vi "Get MeasLink API Path.vi"(11 "error in (no error)":errorcluster) -> (6 "MeasLink API Paths":path[](array[path]), 15 "error out":errorcluster)   [LabVIEW 2021, in "Path Functions.lvlib"]
uses:
  Path Functions.lvlib
  Converter Reusables/Converter Reusables.lvlib
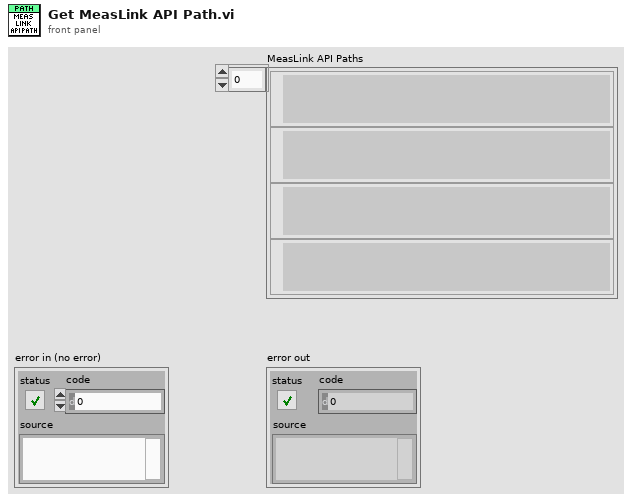
[diagram p1: front panel]
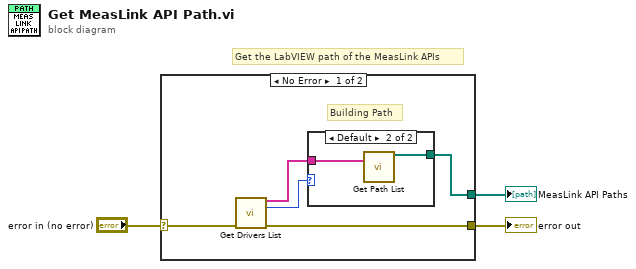
[diagram p0: block diagram]
diagram:
  # "Get the LabVIEW path of the MeasLink APIs"
  n1 = case shown="No Error" "error in (no error)" {
    selector: "error in (no error)" -> [w4 w11]
    tunnel: [w8 _] -> w3
    tunnel: [w6 w11] -> w2
    frame No Error {
      # "Building Path"
      n2 = call "Get Drivers List.vi"("error in (no error)"=w4) -> ("Drivers List Out"=w7:string[], "Total Driver List"=w5:i32, "error out"=w6:errorcluster)  [unwired: 9 in, 3 out]
      n3 = case shown="Default" w5 {
        tunnel: [_ w10] -> w8
        tunnel: w7 -> [_ w9]
        frame 0 {
        }
        frame Default {
          n4 = call "Get Path List.vi"("Drivers List"=w9) -> ("APIs Path"=w10:path[])  [unwired: 14 in]
        }
      }
    }
    frame Error {
    }
  }
  "MeasLink API Paths" <- w3
  "error out" <- w2
